vi "Configure Efficiency Equation.vi"(7 "Formula Number (1)":i32=1 min=1 max=4 step=1, 8 "error in (no error)":errorcluster, 9 "Denominator (0: Off)":i32(ring) items=["Off", "Active Power 1", "Active Power 2", "Active Power 3", "Active Power 4", "Active Power 5", "Active Power 6", "Active Power Sigma A", "Active Power Sigma B", "Active Power Sigma C", "Pm", "User Define 1", "User Define 2"], 10 "Numerator (0: Off)":i32(ring) items=["Off", "Active Power 1", "Active Power 2", "Active Power 3", "Active Power 4", "Active Power 5", "Active Power 6", "Active Power Sigma A", "Active Power Sigma B", "Active Power Sigma C", "Pm", "User Define 1", "User Define 2"], 11 "VISA resource name":refnum<visa-resource-name>) -> (0 "error out":errorcluster, 3 "VISA resource name out":refnum<visa-resource-name>)   [LabVIEW 2021, in "Yokogawa WT1800 Series.lvlib"]
doc: "Create an efficiency equation by combining measurement function symbols. \nThe WT1800 can determine the energy conversion efficiency of the device using the \nnumeric values of the measurement functions."
uses:
  <instrlib>/Yokogawa WT1800 Series/Yokogawa WT1800 Series.lvlib
panel:
  # "X 100 [%]"
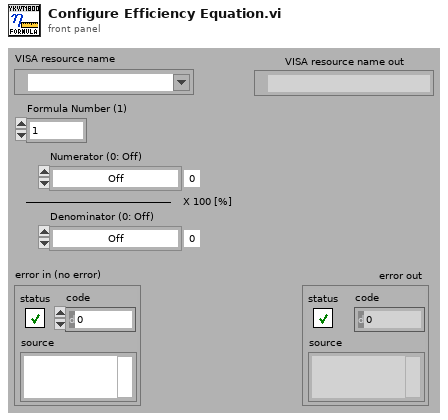
[diagram p1: front panel]
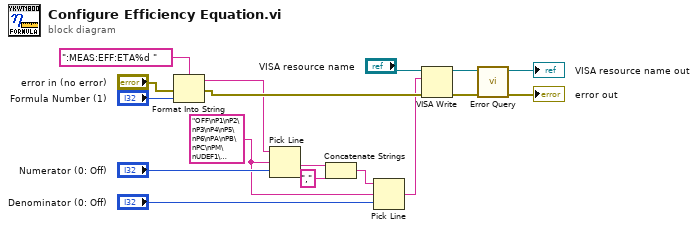
[diagram p0: block diagram]
diagram:
  w6 = "OFF\nP1\nP2\nP3\nP4\nP5\nP6\nPA\nPB\nPC\nPM\nUDEF1\nUDEF2" ("複数行文字列")
  n1 = Format Into String ("文字列にフォーマット")(format string=":MEAS:EFF:ETA%d " ("形式文字列"), error in="error in (no error)", "Formula Number (1)") -> (resulting string=w8:string, error out=w11:errorcluster)  [unwired: 1 in]
  n2 = Pick Line ("ライン選択")(string ("")=w8, multi-line string=w6, line index="Numerator (0: Off)") -> (output string=w3:string)
  n3 = Concatenate Strings(w3, "," ("文字列")) -> (w2:string)
  n4 = Pick Line ("ライン選択")(string ("")=w2, multi-line string=w6, line index="Denominator (0: Off)") -> (output string=w5:string)
  n5 = VISA Write ("VISA書き込み")(VISA resource name="VISA resource name", write buffer=w5, error in (no error)=w11) -> (VISA resource name out=w17:refnum<visa-resource-name>, error out=w16:errorcluster)  [unwired: 1 out]
  n6 = call <instrlib>:"Error Query.vi"("error in (no error)"=w16, "VISA resource name"=w17) -> ("error out"=→"error out":errorcluster, "VISA resource name out"=→"VISA resource name out":refnum<visa-resource-name>)  [unwired: 6 in, 2 out]
